vi "Set Producer Values.vi"(1 "Producer Ch":T1[](array[typedef])=[{"OutputEnable.STS"=0, "ControlMode.STS"=0, "Actual Value.AV"=0.0}], 2 "Producer Control":T2, 8 "error in":errorcluster, 11 "Device Cluster.lvclass in":refnum<class "Device Cluster.lvclass">) -> (0 "error out":errorcluster, 3 "Device Cluster.lvclass out":refnum<class "Device Cluster.lvclass">)   [LabVIEW 2023, in "Device Cluster.lvclass"]
uses:
  Device Cluster.lvclass
  Producer Control.ctl
  Producer Ch.ctl
  Device Cluster.lvclass/Device Cluster.ctl
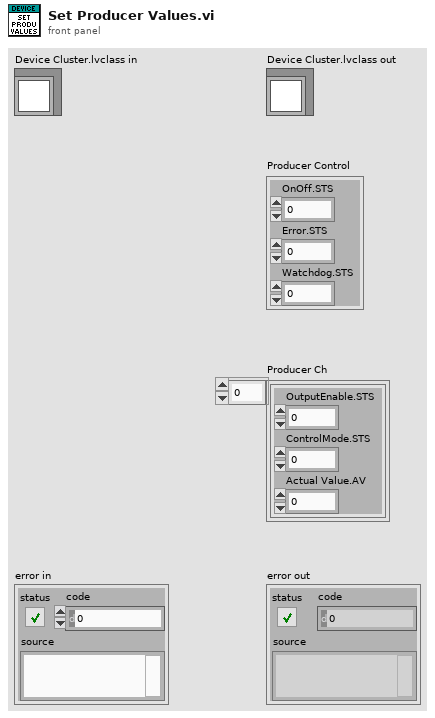
[diagram p1: front panel]
types:
  T1 = typedef "Device Cluster.lvclass/Producer Ch.ctl" = cluster{"OutputEnable.STS":i32, "ControlMode.STS":u16, "Actual Value.AV":dbl}
  T2 = typedef "Device Cluster.lvclass/Producer Control.ctl" = cluster{"OnOff.STS":i32, "Error.STS":i32, "Watchdog.STS":i32}
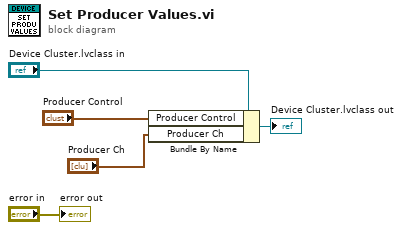
[diagram p0: block diagram]
diagram:
  n1 = Bundle By Name(cluster="Device Cluster.lvclass in", "Producer Control"="Producer Control", "Producer Ch"="Producer Ch") -> (→"Device Cluster.lvclass out":refnum<class "Device Cluster.lvclass">)
  "error out" <- "error in"
